vi "I32 To String (Fix Length).vi"(1 "I32":i32, 6 "Length (Nb Char)":u8) -> (15 "String OUT":string)   [LabVIEW 2020, in "Generic Utilities.lvclass"]
uses:
  Generic Utilities.lvclass
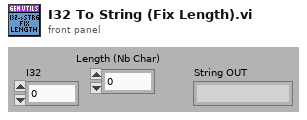
[diagram p1: front panel]
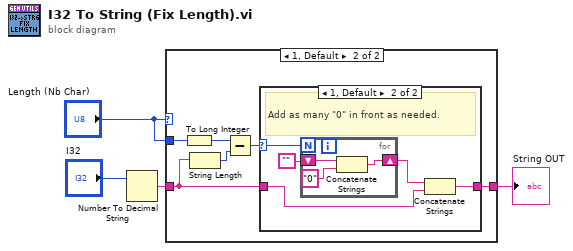
[diagram p0: block diagram]
diagram:
  n1 = Number To Decimal String(number="I32") -> (decimal integer string=w2:string)  [unwired: 1 in]
  n2 = case shown="1, Default" "Length (Nb Char)" {
    tunnel: [w5 w7] -> w3
    tunnel: w2 -> [w5 w6]
    tunnel: "Length (Nb Char)" -> [_ w11]
    frame 0 {
      # "Do Nothing"
    }
    frame 1, Default {
      n3 = To Long Integer(number=w11) -> (32bit integer=w9:i32)
      n4 = String Length(string=w6) -> (length=w10:i32)
      n5 = Subtract(x=w9, y=w10) -> (x-y=w8:i32)
      n6 = case shown="1, Default" w8 {
        selector: w8 -> [_ w17]
        tunnel: [w12 w15] -> w7
        tunnel: w6 -> [w12 w13]
        frame ..0 {
          # "The string lenght is equal or greate, so do nothing"
        }
        frame 1, Default {
          # "Add as many \"0\" in front as needed."
          n7 = for {
            N: w17 -> [_]
            shift-right: [w19] -> w14
            shift-left: "" -> [w20]
            n8 = Concatenate Strings(w20, "0") -> (w19:string)
          }
          n9 = Concatenate Strings(w14, w13) -> (w15:string)
        }
      }
    }
  }
  "String OUT" <- w3
